vi "active object queue_Create.vi"(0 "reference in":refnum<class "active object queue.lvclass">, 5 "error in (no error)":errorcluster) -> (14 "reference out":refnum<class "active object queue.lvclass">, 19 "error out":errorcluster)   [LabVIEW 2019, in "active object queue.lvclass"]
uses:
  active object queue.lvclass
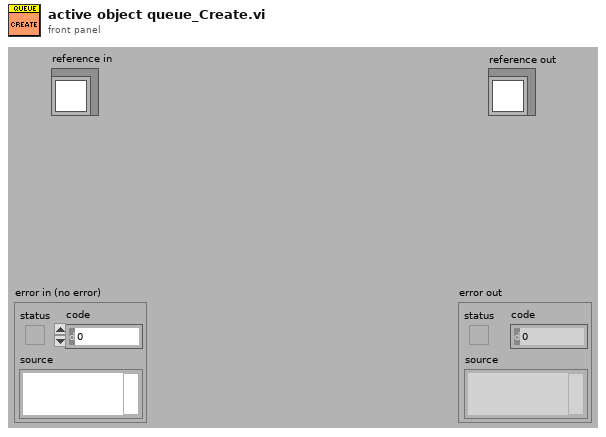
[diagram p1: front panel]
types:
  T1 = typedef "active object queue.lvclass/ObjectAttributes.ctl" = cluster{"Attribute1":dbl, "Status":bool}
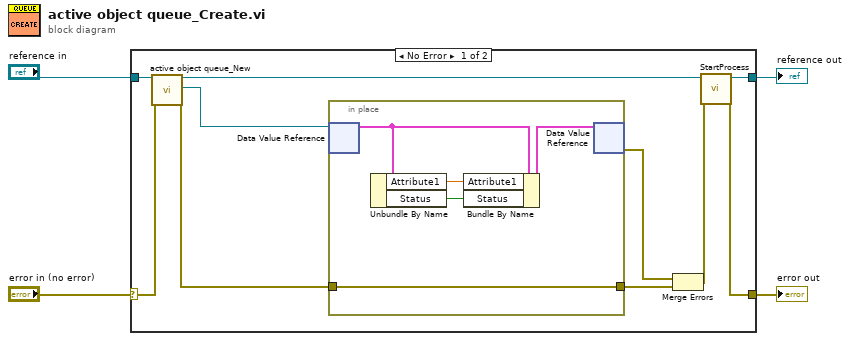
[diagram p0: block diagram]
diagram:
  n1 = case shown="No Error" "error in (no error)" {
    selector: "error in (no error)" -> [w13 w21]
    tunnel: [w5 w21] -> w3
    tunnel: "reference in" -> [w14 w20]
    tunnel: [w7 w20] -> w1
    frame No Error {
      n2 = call "active object queue_New.vi"("reference in"=w14, "error in (no error)"=w13) -> ("reference out"=w8:refnum<class "active object queue.lvclass">, "DVRRefOut"=w11:refnum<data-value>, "error out"=w10:errorcluster)  [unwired: 14 in, 1 out]
      n3 = in-place {
        in-place-border: w10 -> [w16]
        in-place-border: [w16] -> w9
        n4 = in-place-dvr #1(w11) -> (w18:T1)  [unwired: 1 out]
        n5 = Unbundle By Name(w18) -> ("Attribute1"=w17:dbl, "Status"=w15:bool)
        n6 = Bundle By Name(cluster=w18, "Attribute1"=w17, "Status"=w15) -> (w19:T1)
        n7 = in-place-dvr #1(w19) -> (w12:errorcluster)  [unwired: 1 out]
      }
      n8 = Merge Errors(w12, w9) -> (w6:errorcluster)
      n9 = call "StartProcess.vi"("reference in"=w8, "error in (no error)"=w6) -> ("reference out"=w7:refnum<class "active object queue.lvclass">, "error out"=w5:errorcluster)  [unwired: 16 in]
    }
    frame Error {
    }
  }
  "error out" <- w3
  "reference out" <- w1
